vi "test-cubic-spline-03.vi"() -> ()   [LabVIEW 2019]
uses:
  <vilib>/Rock Robotics/WPI/ThirdParty/JAS_Junk/TrajLib/POSEwCURVATURE.ctl
  <vilib>/Rock Robotics/WPI/ThirdParty/JAS_Junk/TrajLib/POSE2D.ctl
  <vilib>/Rock Robotics/WPI/ThirdParty/JAS_Junk/TrajLib/TRANSLATION2D.ctl
  <vilib>/Rock Robotics/WPI/ThirdParty/JAS_Junk/TrajLib/ROTATION2D.ctl
  <vilib>/Rock Robotics/WPI/ThirdParty/JAS_Junk/TrajLib/Rotation_CreateAngle.vi
  <vilib>/Rock Robotics/WPI/ThirdParty/JAS_Junk/TrajLib/Util_CalcDist.vi
  <vilib>/Rock Robotics/WPI/ThirdParty/JAS_Junk/TrajLib/Trajectory_Library.lvlib
panel:
  out "All Interior \nwayPoints\nFound (True)":bool
  out "end rot = 0":dbl
  out "end y = 0":dbl
  out "end x = 0":dbl
  out "start rot = 0":dbl
  out "start y = 0":dbl
  out "start x = 0":dbl
  out "max dtheta < 0.0872":dbl
  out "max dy < 0.00127":dbl
  out "max dx  < 0.127":dbl
  out "Overall Error":errorcluster
  out "Elements":i32
  out "Create Spline Error":errorcluster
  out "SplinePoses\nWCurve":T1[](array[typedef]) {"POSE"."ROTATION"."SIN" format="%13.4f"; "POSE"."ROTATION"."COS" format="%13.4f"; "POSE"."ROTATION"."VALUE" format="%13.4f"; "POSE"."TRANSLATION"."Y" format="%14.3f"; "POSE"."TRANSLATION"."X" format="%14.3f"}
  out "Elapsed Time":dbl
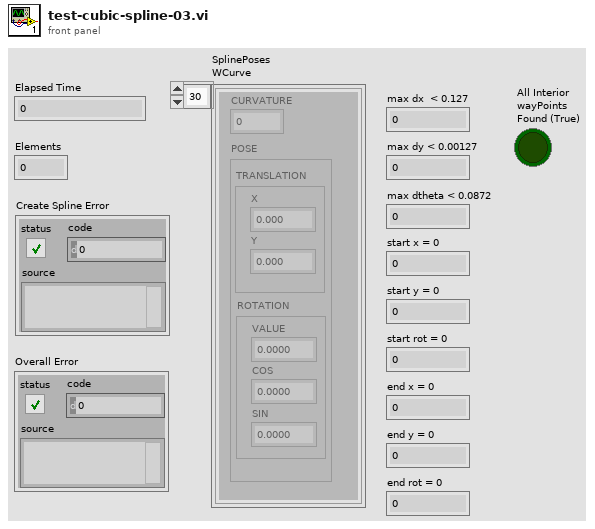
[diagram p1: front panel]
types:
  T1 = typedef "Trajectory_Library.lvlib/POSEwCURVATURE.ctl" = cluster{"CURVATURE":dbl, "POSE":T2}
  T2 = typedef "Trajectory_Library.lvlib/POSE2D.ctl" = cluster{"TRANSLATION":T3, "ROTATION":T4}
  T3 = typedef "Trajectory_Library.lvlib/TRANSLATION2D.ctl" = cluster{"X":dbl, "Y":dbl}
  T4 = typedef "Trajectory_Library.lvlib/ROTATION2D.ctl" = cluster{"VALUE":dbl, "COS":dbl, "SIN":dbl}
  T5 = typedef "Trajectory_Library.lvlib/SPLINE_CTRL_VECTOR.ctl" = cluster{"Xs":dbl[], "Ys":dbl[]}
  T6 = typedef "Trajectory_Library.lvlib/SPLINE.ctl" = cluster{"Degree":i32, "Coefficients":T7}
  T7 = typedef "NI_Matrix.lvlib/RealMatrix.ctl" = dbl[][]
  T8 = typedef "Trajectory_Library.lvlib/TWIST2D.ctl" = cluster{"dX":dbl, "dY":dbl, "dTHETA":dbl}
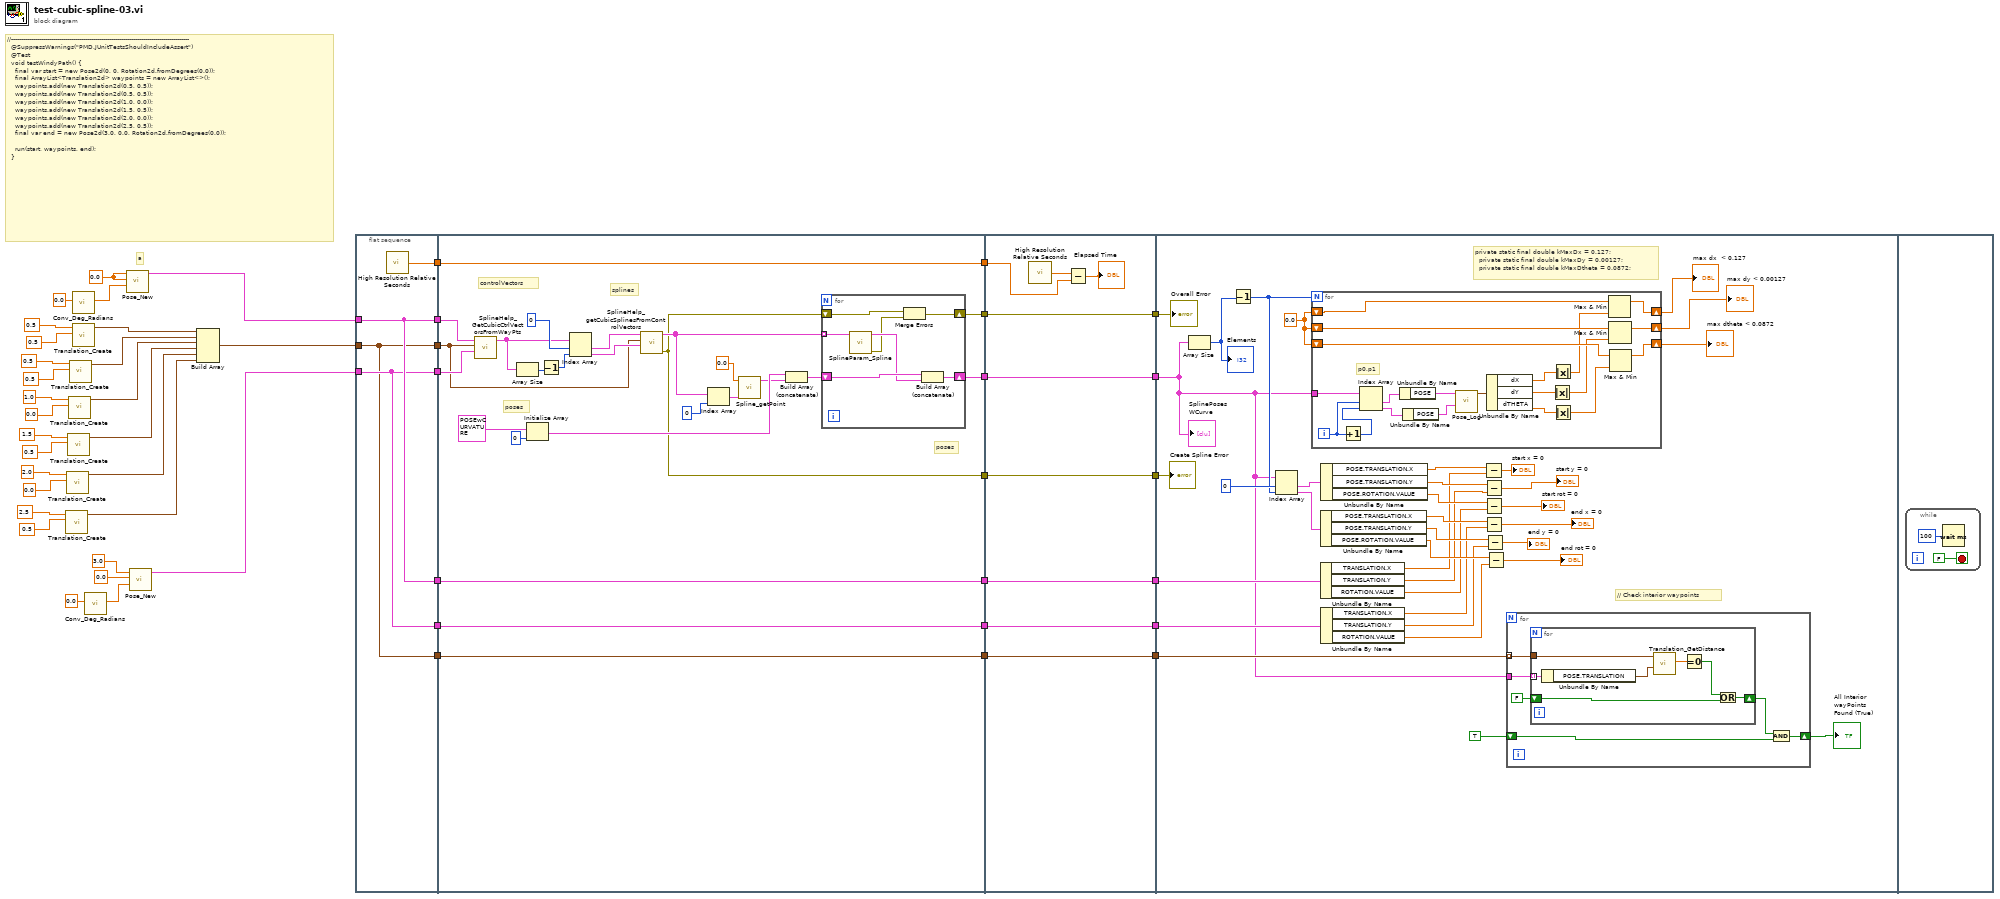
[diagram p0: block diagram]
diagram:
  w24 = 0.0 ("X")
  # "a"
  # "//-----------------------------------------------------------------------------------------\n  @SuppressWarnings(\"PMD.JUnitTestsShouldIncludeAssert\")\n  @Test\n  void testWindyPath() {\n    final var start = new Pose2d(0, 0, Rotation2d.fromDegrees(0.0));\n    final ArrayList<Translation2d> waypoints = new ArrayList<>();\n    waypoints.add(new Translation2d(0.5, 0.5));\n    waypoints.add(new Translation2d(0.5, 0.5));\n    waypoints.add(new Translation2d(1.0, 0.0));\n    waypoints.add(new Translation2d(1.5, 0.5));\n    waypoints.add(new Translation2d(2.0, 0.0));\n    waypoints.add(new Translation2d(2.5, 0.5));\n    final var end = new Pose2d(3.0, 0.0, Rotation2d.fromDegrees(0.0));\n\n    run(start, waypoints, end);\n  }"
  n1 = call <vilib>:"Translation_Create.vi"("Y"=0.5, "X"=2.5) -> ("TRANSLATION"=w1:T3)  [unwired: 9 in]
  n2 = call <vilib>:"Translation_Create.vi"("Y"=0.0, "X"=2.0) -> ("TRANSLATION"=w2:T3)  [unwired: 9 in]
  n3 = call <vilib>:"Translation_Create.vi"("Y"=0.5, "X"=1.5) -> ("TRANSLATION"=w3:T3)  [unwired: 9 in]
  n4 = call <vilib>:"Translation_Create.vi"("Y"=0.0, "X"=1.0) -> ("TRANSLATION"=w4:T3)  [unwired: 9 in]
  n5 = call <vilib>:"Translation_Create.vi"("Y"=0.5, "X"=0.5) -> ("TRANSLATION"=w5:T3)  [unwired: 9 in]
  n6 = call <vilib>:"Conv_Deg_Radians.vi"("Degress"=0.0) -> ("Radians"=w23:dbl)  [unwired: 10 in]
  n7 = call <vilib>:"Translation_Create.vi"("Y"=0.5, "X"=0.5) -> ("TRANSLATION"=w20:T3)  [unwired: 9 in]
  n8 = call <vilib>:"Conv_Deg_Radians.vi"("Degress"=0.0) -> ("Radians"=w16:dbl)  [unwired: 10 in]
  n9 = call <vilib>:"Pose_New.vi"("Heading"=w23, "Y"=w24, "X"=w24) -> ("out POSe"=w46:T2)  [unwired: 8 in]
  n10 = call <vilib>:"Pose_New.vi"("Heading"=w16, "Y"=0.0, "X"=3.0) -> ("out POSe"=w43:T2)  [unwired: 8 in]
  n11 = Build Array(w20, w5, w4, w3, w2, w1) -> (w21:T3[])
  n12 = flat-sequence {
    tunnel: w46 -> [w51]
    tunnel: [w51] -> w45
    tunnel: w21 -> [w49]
    tunnel: [w49] -> w44
    tunnel: w43 -> [w50]
    tunnel: [w50] -> w42
    tunnel: [w52] -> w41
    tunnel: [w51] -> w33
    tunnel: [w50] -> w30
    tunnel: [w49] -> w25
    tunnel: w45 -> [w77]
    tunnel: w44 -> [w69]
    tunnel: w42 -> [w76]
    tunnel: [w68] -> w40
    tunnel: w41 -> [w68]
    tunnel: [w58] -> w39
    tunnel: [w57] -> w37
    tunnel: [w56] -> w35
    tunnel: w33 -> [w55]
    tunnel: [w55] -> w32
    tunnel: w30 -> [w54]
    tunnel: [w54] -> w29
    tunnel: [w53] -> w26
    tunnel: w25 -> [w53]
    tunnel: w40 -> [w93]
    tunnel: w39 -> [w92]
    tunnel: [w92] -> w38
    tunnel: w37 -> [w91]
    tunnel: [w91] -> w36
    tunnel: w35 -> [w90]
    tunnel: [w90] -> w34
    tunnel: w32 -> [w87]
    tunnel: [w87] -> w31
    tunnel: w29 -> [w86]
    tunnel: [w86] -> w28
    tunnel: [w85] -> w27
    tunnel: w26 -> [w85]
    tunnel: w38 -> [w96]
    tunnel: w36 -> [w128]
    tunnel: w34 -> [w127]
    tunnel: w31 -> [w121]
    tunnel: w28 -> [w120]
    tunnel: w27 -> [w97]
    frame #0 {
      n13 = call <vilib>:"High Resolution Relative Seconds.vi"() -> ("relative seconds"=w52:dbl)
    }
    frame #1 {
      # "poses"
      # "poses"
      # "splines"
      # "controlVectors"
      n14 = call <vilib>:"SplineHelp_GetCubicCtrlVectorsFromWayPts.vi"("Enging POSE"=w76, "Interior WAYPOINTS"=w69, "Starting POSE"=w77) -> ("SplineControlVectors"=w73:T5[])  [unwired: 8 in]
      n15 = Array Size(array=w73) -> (size(s)=w74:i32)
      n16 = Initialize Array(T1 {"CURVATURE"=0.0, "POSE"={"TRANSLATION"={"X"=0.0, "Y"=0.0}, "ROTATION"={"VALUE"=0.0, "COS"=1.0, "SIN"=0.0}}} ("POSEwCURVATURE"), 0 ("dimension size")) -> (w62:T1[])
      n17 = Decrement(x=w74) -> (x-1=w72:i32)
      n18 = Index Array(array=w73, index #1=0 ("index"), index #2=w72) -> (element #1=w71:T5, element #2=w70:T5)
      n19 = call <vilib>:"SplineHelp_getCubicSplinesFromControlVectors.vi"("endCtrlVector"=w70, "InternalWaypoints"=w69, "startCtrlVector"=w71) -> ("error out"=w57:errorcluster, "splines"=w59:T6[])  [unwired: 3 in, 4 out]
      n20 = Index Array(array=w59, index=0) -> (element=w64:T6)
      n21 = call <vilib>:"Spline_getPoint.vi"("inputSPLINE"=w64, "Time"=0.0) -> ("POSEwCURVATURE"=w61:T1)  [unwired: 9 in]
      n22 = Build Array (concatenate)(w62, w61) -> (w60:T1[])
      n23 = for {
        shift-right: [w81] -> w58
        shift-left: w60 -> [w83]
        tunnel: w59 -> [w84] mode=indexing
        shift-right: [w79] -> w56
        shift-left: w57 -> [w80]
        n24 = call <vilib>:"SplineParam_Spline.vi"("inputSPLINE"=w84) -> ("error out"=w78:errorcluster, "outputPOSEwCURVATURE"=w82:T1[])  [unwired: 9 in]
        n25 = Merge Errors(w80, w78) -> (w79:errorcluster)
        n26 = Build Array (concatenate)(w83, w82) -> (w81:T1[])
      }
    }
    frame #2 {
      n27 = call <vilib>:"High Resolution Relative Seconds.vi"() -> ("relative seconds"=w88:dbl)
      n28 = Subtract(x=w88, y=w93) -> (x-y=→"Elapsed Time":dbl)
    }
    frame #3 {
      w125 = 0.0
      # "// Check interior waypoints"
      # "private static final double kMaxDx = 0.127;\n  private static final double kMaxDy = 0.00127;\n  private static final double kMaxDtheta = 0.0872;"
      n29 = Array Size(array=w96) -> (size(s)=w126:i32)
      "Elements" <- w126
      n30 = Decrement(x=w126) -> (x-1=w118:i32)
      n31 = Index Array(array=w96, index #1=0 ("index"), index #2=w118) -> (element #1=w117:T1, element #2=w116:T1)
      n32 = for {
        N: w118 -> [_]
        tunnel: w96 -> [w159]
        shift-right: [w150] -> w124
        shift-left: w125 -> [w147]
        shift-right: [w148] -> w122
        shift-left: w125 -> [w145]
        shift-right: [w149] -> w123
        shift-left: w125 -> [w146]
        i -> [w161]
        # "p0,p1"
        n33 = Increment(x=w161) -> (x+1=w160:i32)
        n34 = Index Array(array=w159, index #1=w161, index #2=w160) -> (element #1=w158:T1, element #2=w157:T1)
        n35 = Unbundle By Name(w158) -> ("POSE"=w156:T2)
        n36 = Unbundle By Name(w157) -> ("POSE"=w155:T2)
        n37 = call <vilib>:"Pose_Log.vi"("end POSE"=w155, "in POSE"=w156) -> ("out TWIST"=w154:T8)  [unwired: 9 in]
        n38 = Unbundle By Name(w154) -> ("dX"=w151:dbl, "dY"=w152:dbl, "dTHETA"=w153:dbl)
        n39 = Absolute Value(x=w152) -> (abs(x)=w143:dbl)
        n40 = Absolute Value(x=w151) -> (abs(x)=w144:dbl)
        n41 = Absolute Value(x=w153) -> (abs(x)=w142:dbl)
        n42 = Max & Min(x=w147, y=w144) -> (max(x,y)=w150:dbl)  [unwired: 1 out]
        n43 = Max & Min(x=w146, y=w143) -> (max(x,y)=w149:dbl)  [unwired: 1 out]
        n44 = Max & Min(x=w145, y=w142) -> (max(x,y)=w148:dbl)  [unwired: 1 out]
      }
      "max dx  < 0.127" <- w124
      "max dy < 0.00127" <- w123
      "max dtheta < 0.0872" <- w122
      n45 = Unbundle By Name(w116) -> ("POSE.TRANSLATION.X"=w112:dbl, "POSE.TRANSLATION.Y"=w111:dbl, "POSE.ROTATION.VALUE"=w110:dbl)
      n46 = Unbundle By Name(w121) -> ("TRANSLATION.X"=w109:dbl, "TRANSLATION.Y"=w108:dbl, "ROTATION.VALUE"=w107:dbl)
      n47 = Unbundle By Name(w117) -> ("POSE.TRANSLATION.X"=w115:dbl, "POSE.TRANSLATION.Y"=w114:dbl, "POSE.ROTATION.VALUE"=w113:dbl)
      n48 = Unbundle By Name(w120) -> ("TRANSLATION.X"=w106:dbl, "TRANSLATION.Y"=w105:dbl, "ROTATION.VALUE"=w104:dbl)
      n49 = Subtract(x=w115, y=w109) -> (x-y=→"start x = 0":dbl)
      n50 = Subtract(x=w114, y=w108) -> (x-y=→"start y = 0":dbl)
      n51 = Subtract(x=w113, y=w107) -> (x-y=→"start rot = 0":dbl)
      n52 = Subtract(x=w112, y=w106) -> (x-y=→"end x = 0":dbl)
      n53 = Subtract(x=w111, y=w105) -> (x-y=→"end y = 0":dbl)
      n54 = Subtract(x=w110, y=w104) -> (x-y=→"end rot = 0":dbl)
      n55 = for {
        tunnel: w97 -> [w129] mode=indexing
        tunnel: w96 -> [w134]
        shift-right: [w133] -> w94
        shift-left: TRUE -> [w132]
        n56 = for {
          tunnel: w134 -> [w138] mode=indexing
          shift-right: [w141] -> w130
          shift-left: FALSE -> [w140]
          tunnel: w129 -> [w139]
          n57 = Unbundle By Name(w138) -> ("POSE.TRANSLATION"=w137:T3)
          n58 = call <vilib>:"Translation_GetDistance.vi"("other Translation"=w137, "In Translation"=w139) -> ("Distance"=w136:dbl)  [unwired: 9 in]
          n59 = Equal To 0?(x=w136) -> (x = 0?=w135:bool)
          n60 = Or(x=w135, y=w140) -> (x .or. y?=w141:bool)
        }
        n61 = And(x=w130, y=w132) -> (x .and. y?=w133:bool)
      }
      "All Interior \nwayPoints\nFound (True)" <- w94
      "SplinePoses\nWCurve" <- w96
      "Create Spline Error" <- w128
      "Overall Error" <- w127
    }
    frame #4 {
      n62 = while {
        stop <- FALSE stop-if-true
        n63 = Wait (ms)(milliseconds to wait=u32 100) -> ()  [unwired: 1 out]
      }
    }
  }
